vi "Pos_Move Box to Point.vi"(8 "Error":errorcluster, 9 "Point":T2, 10 "Position":T3, 11 "Window":T1) -> (0 "Error Out":errorcluster, 3 "Window Out":T1)   [LabVIEW 2024]
uses:
  TypeDefs_Utility/ENUM RB_Pos_Quadrant Position.ctl
  TypeDefs_Utility/Cluster_Top Left position.ctl
  <vilib>/Utility/miscctls.llb/LVRectTypeDef.ctl
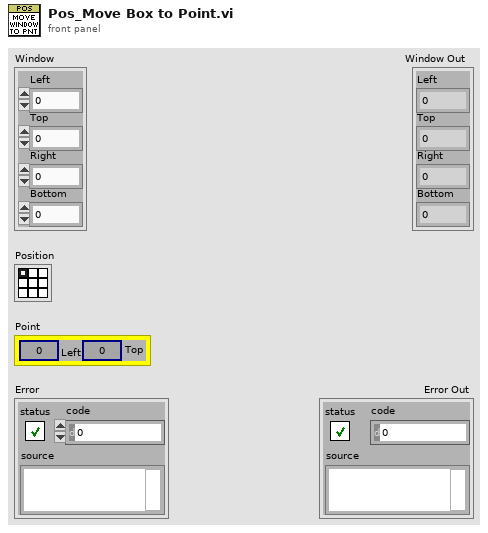
[diagram p1: front panel]
types:
  T1 = typedef "LVRectTypeDef.ctl" = cluster{"Left":i16, "Top":i16, "Right":i16, "Bottom":i16}
  T2 = typedef "Cluster_Top Left position.ctl" = cluster{"Left":i32, "Top":i32}
  T3 = typedef "ENUM RB_Pos_Quadrant Position.ctl" = enum32{"LFT-TOP", "MID-TOP", "RGT-TOP", "LFT-CTR", "MID-CTR", "RGT-CTR", "LFT-BOT", "MID-BOT", "RGT-BOT"}
  T4 = typedef "Cluster_Pos_Top Left position.ctl" = cluster{"Left":i16, "Top":i16}
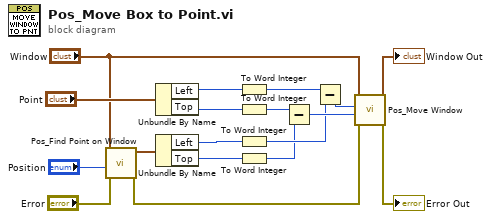
[diagram p0: block diagram]
diagram:
  n1 = call "Pos_Find Point on Window.vi"("Error"="Error", "Position"="Position", "Window"="Window") -> ("Error Out"=w11:errorcluster, "Point Out"=w13:T4)  [unwired: 7 in]
  n2 = Unbundle By Name("Point") -> ("Left"=w10:i32, "Top"=w7:i32)
  n3 = Unbundle By Name(w13) -> ("Left"=w9:i16, "Top"=w6:i16)
  n4 = To Word Integer(number=w10) -> (16bit integer=w4:i16)
  n5 = To Word Integer(number=w7) -> (16bit integer=w3:i16)
  n6 = To Word Integer(number=w9) -> (16bit integer=w2:i16)
  n7 = To Word Integer(number=w6) -> (16bit integer=w1:i16)
  n8 = Subtract(x=w3, y=w1) -> (x-y=w5:i16)
  n9 = Subtract(x=w4, y=w2) -> (x-y=w8:i16)
  n10 = call "Pos_Move Window.vi"("Error"=w11, "Down"=w5, "Right"=w8, "Window"="Window") -> ("Error Out"=→"Error Out":errorcluster, "Window Out"=→"Window Out":T1)  [unwired: 6 in]
